vi "DI Coil UI.vi"(8 "error in (no error)":errorcluster, 11 "Node Ptr":T2 format="%.0x") -> (0 "error out":errorcluster)   [LabVIEW 2015, in "Modbus Master System Explorer.lvlib"]
uses:
  Modbus Master System Explorer.lvlib
  <vilib>/NI Veristand/Custom Device API/Custom Device Item Ref.ctl
  SubVIs/Radix.ctl
  <vilib>/NI VeriStand/Custom Device API/Custom Device API.lvlib
panel:
  in  "Radix":T1
  in  "Valid?":string
  in  "Mapping":u16
  in  "Header":cluster{"Section Name":string}={"Section Name"="Discrete Input Settings"}
  in  "Description":string
  in  "Name":string
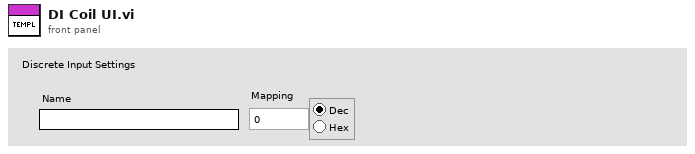
[diagram p1: front panel]
types:
  T1 = typedef "Modbus Master System Explorer.lvlib/Radix.ctl" = enum32{"Decimal", "Hexidecimal"}
  T2 = typedef "Custom Device API.lvlib/Custom Device Item Ref.ctl" = u64
  T3 = typedef "Custom Device API.lvlib/Custom Device Item Info.ctl" = cluster{"Name":string, "Is Channel":bool, "GUID":string, "Is Waveform":bool}
  T4 = typedef "Custom Device API.lvlib/Custom Device Commands.ctl" = enum16{"Default", "Item renamed", "Shutdown", "Dynamic button pressed"}
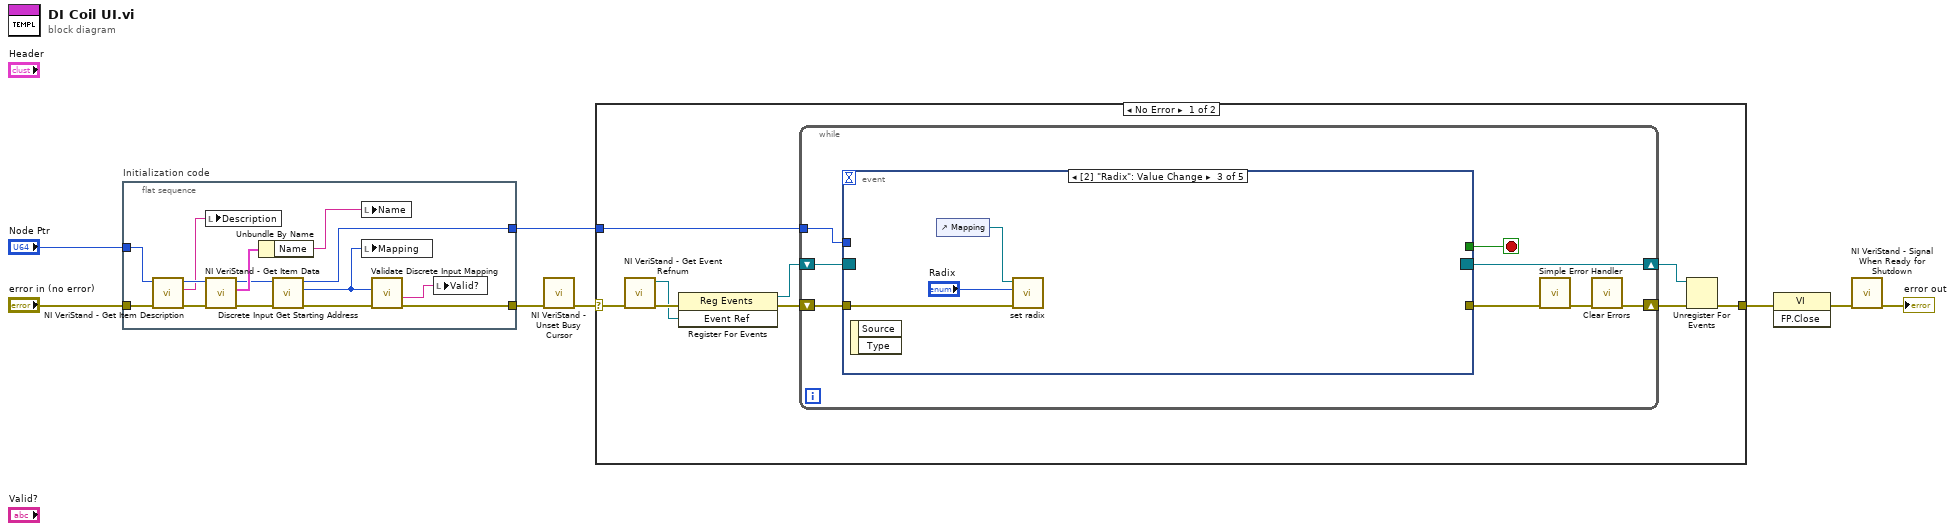
[diagram p0: block diagram]
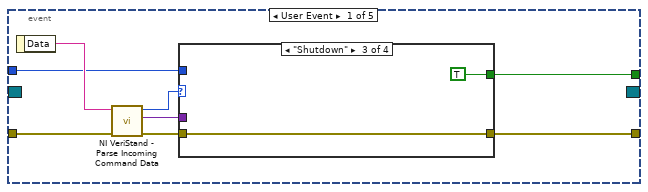
[diagram p2: hidden frame]
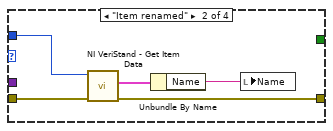
[diagram p4: hidden frame]
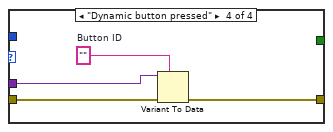
[diagram p5: hidden frame]
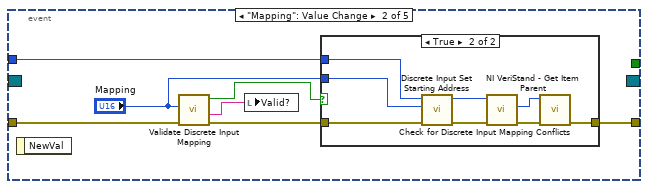
[diagram p6: hidden frame]
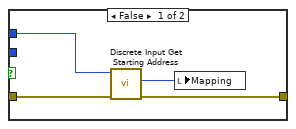
[diagram p7: hidden frame]
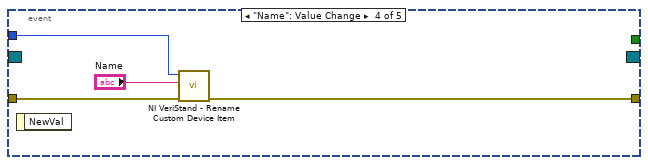
[diagram p8: hidden frame]
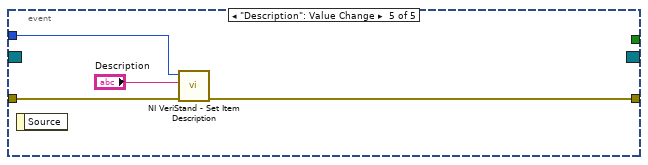
[diagram p9: hidden frame]
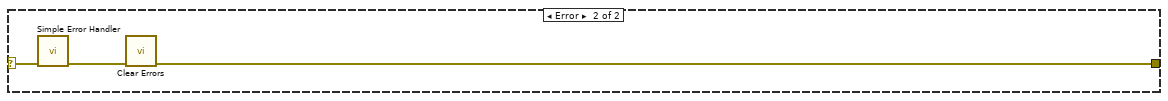
[diagram p10: hidden frame]
diagram:
  n1 = flat-sequence "Initialization code" {
    tunnel: "error in (no error)" -> [w21]
    tunnel: "Node Ptr" -> [w20]
    tunnel: [w14] -> w4
    tunnel: [w9] -> w1
    frame #0 {
      n2 = call <vilib>:"NI VeriStand - Get Item Description.vi"("error in (no error)"=w21, "Item Ref in"=w20) -> ("error out"=w18:errorcluster, "Description"=w19:string, "Item Ref out"=w22:T2)  [unwired: 7 out]
      n3 = local write "Description"(w19) -> ()
      n4 = call <vilib>:"NI VeriStand - Get Item Data.vi"("error in (no error)"=w18, "Item Ref in"=w22) -> ("error out"=w11:errorcluster, "Item Info"=w17:T3, "Item Ref out"=w10:T2)  [unwired: 7 out]
      n5 = Unbundle By Name(w17) -> ("Name"=w16:string)
      n6 = call "Discrete Input Get Starting Address.vi"("error in (no error)"=w11, "Item Ref in"=w10) -> ("error out"=w12:errorcluster, "Starting Address"=w13:u16, "Item Ref out"=w9:T2)  [unwired: 7 in]
      n7 = local write "Name"(w16) -> ()
      n8 = local write "Mapping"(w13) -> ()
      n9 = call "Validate Discrete Input Mapping.vi"("error in (no error)"=w12, "Mapping"=w13) -> ("error out"=w14:errorcluster, "Status Message"=w15:string)  [unwired: 7 in, 1 out]
      n10 = local write "Valid?"(w15) -> ()
    }
  }
  n11 = call <vilib>:"NI VeriStand - Unset Busy Cursor.vi"("error in (no error)"=w4) -> ("error out"=w3:errorcluster)  [unwired: 10 out]
  n12 = case shown="No Error" w3 {
    selector: w3 -> [w23 w92]
    tunnel: [w28 w90] -> w8
    tunnel: w1 -> [w24 _]
    frame No Error {
      n13 = call <vilib>:"NI VeriStand - Get Event Refnum.vi"("error in (no error)"=w23) -> ("error out"=w31:errorcluster, "Event Ref"=w27:refnum<user-event>)  [unwired: 9 out]
      n14 = register-events(error in=w31, w27) -> (reference out=w25:refnum<event-registration>, error out=w26:errorcluster)  [unwired: 1 in]
      n15 = while {
        tunnel: w24 -> [w35]
        shift-right: [w32] -> w29
        shift-left: w26 -> [w38]
        shift-right: [w39] -> w30
        shift-left: w25 -> [w37]
        stop <- w36 stop-if-true
        n16 = event shown="[2] \"Radix\": Value Change" {
          selector: w37 -> [_ _ _ _ _]
          dyn-events: [_ _ _ _ _] -> w39
          timeout: _ -> [_ _ _ _ _]
          tunnel: w38 -> [w47 w62 w79 w85 w88]
          tunnel: [w43 _ _ _ _] -> w36
          tunnel: [w42 w64 _ w84 w87] -> w34
          tunnel: w35 -> [w41 w66 _ w83 w89]
          event User Event {
            n17 = event-data() -> ("Data"=w46:string)  [unwired: 1 out]
            n18 = call <vilib>:"NI VeriStand - Parse Incoming Command Data.vi"("error in (no error)"=w47, "Incoming data"=w46) -> ("error out"=w45:errorcluster, "Outgoing data"=w40:variant, "Action"=w44:T4)  [unwired: 7 out]
            n19 = case shown="\"Shutdown\"" w44 {
              tunnel: w45 -> [w48 w53 w54 w59]
              tunnel: [_ _ TRUE _] -> w43
              tunnel: [w48 w50 w54 w56] -> w42
              tunnel: w41 -> [_ w52 _ _]
              tunnel: w40 -> [_ _ _ w58]
              frame "Default", Default {
              }
              frame "Item renamed" {
                n20 = call <vilib>:"NI VeriStand - Get Item Data.vi"("error in (no error)"=w53, "Item Ref in"=w52) -> ("error out"=w50:errorcluster, "Item Info"=w51:T3)  [unwired: 8 out]
                n21 = Unbundle By Name(w51) -> ("Name"=w49:string)
                n22 = local write "Name"(w49) -> ()
              }
              frame "Shutdown" {
              }
              frame "Dynamic button pressed" {
                w57 = ""  # Button ID
                n23 = Variant To Data(error in=w59, type=w57, Variant=w58) -> (error out=w56:errorcluster)  [unwired: 1 out]
              }
            }
          }
          event "Mapping": Value Change {
            n24 = event-data() -> ()  [unwired: 2 out]
            n25 = call "Validate Discrete Input Mapping.vi"("error in (no error)"=w62, "Mapping"="Mapping") -> ("error out"=w61:errorcluster, "Status Message"=w60:string, "Valid?"=w63:bool)  [unwired: 7 in]
            n26 = local write "Valid?"(w60) -> ()
            n27 = case shown="True" w63 {
              tunnel: w66 -> [w68 w78]
              tunnel: "Mapping" -> [_ w77]
              tunnel: w61 -> [w70 w76]
              tunnel: [w69 w72] -> w64
              frame False {
                n28 = call "Discrete Input Get Starting Address.vi"("error in (no error)"=w70, "Item Ref in"=w68) -> ("error out"=w69:errorcluster, "Starting Address"=w67:u16)  [unwired: 7 in, 1 out]
                n29 = local write "Mapping"(w67) -> ()
              }
              frame True {
                n30 = call "Discrete Input Set Starting Address.vi"("error in (no error)"=w76, "Value"=w77, "Item Ref in"=w78) -> ("error out"=w75:errorcluster, "Item Ref out"=w71:T2)  [unwired: 7 in]
                n31 = call <vilib>:"NI VeriStand - Get Item Parent.vi"("error in (no error)"=w75, "Item Ref in"=w71) -> ("error out"=w73:errorcluster, "Parent Ref"=w74:T2)  [unwired: 6 in, 2 out]
                n32 = call "Check for Discrete Input Mapping Conflicts.vi"("error in (no error)"=w73, "Coiil Group Ref in"=w74) -> ("error out"=w72:errorcluster)  [unwired: 6 in, 3 out]
              }
            }
          }
          event Value Change {
            n33 = event-data() -> ()  [unwired: 3 out]
            n34 = control-ref of="Mapping"() -> (w80:refnum<vi>)
            n35 = call "set radix.vi"("error in (no error)"=w79, "Radix"="Radix", "Digital in"=w80) -> ()  [unwired: 8 in, 1 out]
          }
          event "Name": Value Change {
            n36 = event-data() -> ()  [unwired: 2 out]
            n37 = call <vilib>:"NI VeriStand - Rename Custom Device Item.vi"("error in (no error)"=w85, "New Name"="Name", "Item Ref in"=w83) -> ("error out"=w84:errorcluster)  [unwired: 1 in, 7 out]
          }
          event "Description": Value Change {
            n38 = event-data() -> ()  [unwired: 2 out]
            n39 = call <vilib>:"NI VeriStand - Set Item Description.vi"("error in (no error)"=w88, "Description"="Description", "Item Ref in"=w89) -> ("error out"=w87:errorcluster)  [unwired: 8 out]
          }
        }
        n40 = call <vilib>:"Simple Error Handler.vi"("error in (no error)"=w34) -> ("error out"=w33:errorcluster)  [unwired: 1 in, 7 out]
        n41 = call <vilib>:"Clear Errors.vi"("error in (no error)"=w33) -> ("error out"=w32:errorcluster)  [unwired: 1 in, 5 out]
      }
      n42 = Unregister For Events(event registration refnum=w30, error in=w29) -> (error out=w28:errorcluster)
    }
    frame Error {
      n43 = call <vilib>:"Simple Error Handler.vi"("error in (no error)"=w92) -> ("error out"=w91:errorcluster)  [unwired: 1 in, 7 out]
      n44 = call <vilib>:"Clear Errors.vi"("error in (no error)"=w91) -> ("error out"=w90:errorcluster)  [unwired: 1 in, 5 out]
    }
  }
  n45 = invoke class="VI" method="FP.Close"(error in=w8) -> (error out=w7:errorcluster)  [unwired: 2 in, 2 out]
  n46 = call <vilib>:"NI VeriStand - Signal When Ready for Shutdown.vi"("error in (no error)"=w7) -> ("error out"=→"error out":errorcluster)  [unwired: 10 out]
